vi "Speed Calibration.vi"() -> ()   [LabVIEW 2016]
uses:
  <vilib>/NXT/Block Support/NXT_OutputPort.ctl
  <vilib>/NXT/Dual Mode Library/Motors/Rotation.vi
panel:
  out "x/y":dbl
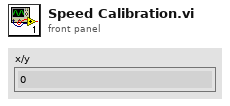
[diagram p1: front panel]
types:
  T1 = typedef "NXT_OutputPort.ctl" = u8
  T2 = typedef "LVHSConnector.ctl" = refnum<class "BrickReference.lvclass">
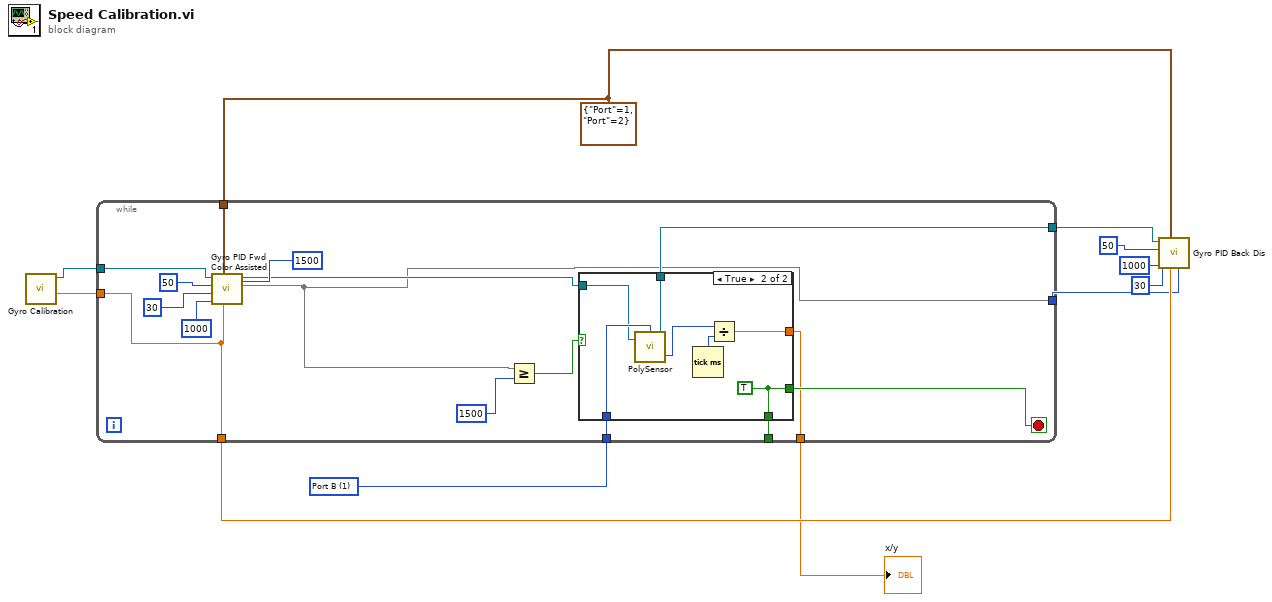
[diagram p0: block diagram]
diagram:
  w8 = cluster{"Port":T1, "Port":T1} {"Port"=1, "Port"=2} ("Motor")
  w2 = T1 1 items=["Port A", "Port B", "Port C", "Port D"] ("Port (Port A)")
  n1 = call "Gyro Calibration.vi"() -> ("Degrees"=w6:sgl, "NXT/EV3"=w7:T2)  [unwired: 7 in, 1 out]
  n2 = while {
    tunnel: w2 -> [w21]
    tunnel: [w19] -> w9
    tunnel: w8 -> [w18]
    tunnel: w7 -> [w17]
    tunnel: w6 -> [w16]
    tunnel: [w16] -> w5
    tunnel: [w14] -> w3
    tunnel: [w13] -> _
    tunnel: [w12] -> w1
    stop <- w20 stop-if-true
    n3 = call "Gyro PID Fwd Color Assisted.vi"(5:1500 ("Threshold to C1"), "Target angle"=w16, "Threshold to Color"=w18, "Threshold to slow"=1000 ("Threshold to De-acc"), "Min. speed"=30 ("De-acc"), "Max. speed"=50 ("Acc"), "EV3 in"=w17) -> (2:w14, "EV3 out"=w15:T2)  [unwired: 3 in]
    n4 = Greater Or Equal?(x=w14, y=1500) -> (x >= y?=w22:bool)
    n5 = case shown="True" w22 {
      tunnel: w21 -> [_ w34]
      tunnel: [_ w33] -> w12
      tunnel: [_ w30] -> w20
      tunnel: [_ w32] -> w19
      tunnel: w15 -> [_ w31]
      tunnel: [_ w30] -> w13
      frame False {
      }
      frame True {
        w30 = TRUE
        n6 = call-poly <vilib>:"PolySensor.vi"("NXT/EV3"=w31, "Port (Port A)"=w34) -> ("Angle of Rotation"=w29:i32, "NXT/EV3"=w32:T2)  [unwired: 1 in]
        n7 = Tick Count (ms)() -> (millisecond timer value=w28:u32)
        n8 = Divide(x=w29, y=w28) -> (x/y=w33:dbl)
      }
    }
  }
  "x/y" <- w1
  n9 = call "Gyro PID Back Dis.vi"(4:w3, "Target angle"=w5, "Threshold to stop"=w8, "Threshold to slow"=1000 ("Threshold to De-acc"), "Min. speed"=30 ("De-acc"), "Max. speed"=50 ("Acc"), "EV3 in"=w9) -> ()  [unwired: 4 in, 1 out]
